vi "Begin.vi"(8 "error in":errorcluster) -> (0 "error out":errorcluster)   [LabVIEW 2017]
doc: "Called before other user functions, this VI is expected to open initial I/O refnums, load in file data, and do all program initialization. Notice that the <B>error out</B> terminal is simply used for data flow. Wiring it to other structures or subVIs ensures that this VI runs first."
uses:
  <vilib>/Rock Robotics/WPI/Solenoid/WPI_SolenoidChannel.ctl
  <vilib>/Rock Robotics/WPI/DriverStation/WPI_DriverStationRobotMode2.ctl
  <vilib>/Rock Robotics/WPI/Joystick/WPI_JoystickDeviceEnum.ctl
  <vilib>/Rock Robotics/SystemInterfaces/spilib/spi_bus.ctl
  Robot Global Data.vi
  <vilib>/Rock Robotics/Network Tables/NT Write String Array.vi
  <vilib>/Rock Robotics/WPI/Solenoid/WPI_SolenoidOpenDouble.vi
  <vilib>/Rock Robotics/WPI/RobotDrive/WPI_RobotDriveOpen4MotorWithExistingMotors.vi
  FIRST-3958-Controls-Library/NavX/navX Library v2/IO/Open/Z900_navX_Open_SPI.vi
  FIRST-3958-Controls-Library/NavX/navX Library v2/navX Library v2.lvlib
panel:
  in  "Reverse Solenoid Channel 2":T1=enum."Solenoid 2"
  in  "Solenoid Channel 2":T1=enum."Solenoid 3"
  in  "Reverse Solenoid Channel":T1
  in  "Solenoid Channel":T1=enum."Solenoid 1"
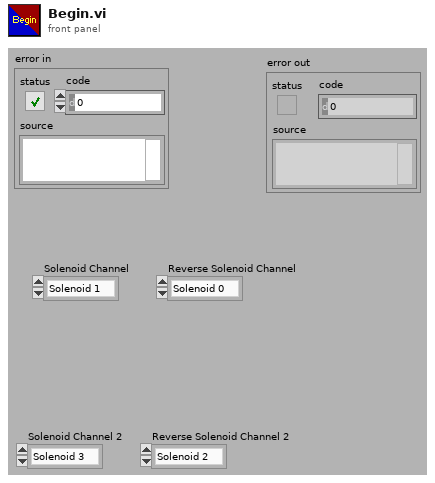
[diagram p1: front panel]
types:
  T1 = typedef "WPI_SolenoidChannel.ctl" = enum8{"Solenoid 0", "Solenoid 1", "Solenoid 2", "Solenoid 3", "Solenoid 4", "Solenoid 5", "Solenoid 6", "Solenoid 7", "Invalid"}
  T2 = typedef "spi_bus.ctl" = enum16{"SPI On-Board, CS0", "SPI On-Board, CS1", "SPI On-Board, CS2", "SPI On-Board, CS3", "SPI MXP", "Invalid"}
  T3 = typedef "WPI_JoystickDeviceEnum.ctl" = enum16{"USB 0", "USB 1", "USB 2", "USB 3", "USB 4", "USB 5"}
  T4 = typedef "WPI_DriverStationRobotMode2.ctl" = enum16{"Autonomous Disabled", "Autonomous Enabled", "Teleop Disabled", "Teleop Enabled", "Disconnected", "Finish", "Test Disabled", "Test Enabled", "Emergency Stopped"}
  T5 = typedef "WPI_MotorControlDeviceRef.ctl" = cluster{"DeviceStatus":errorcluster, "Type":T6, "PWM":cluster{"PWM Channel":T7, "DeadBand":T8}, "CAN":cluster{"Device Number":u8, "SetOutput VI Ref":variant, "GetOutput VI Ref":variant, "Enable VI Ref":variant, "Disable VI Ref":variant, "Data":variant}, "Invert":bool, "DIO PWM":cluster{"PWM \"Enable\" Channel":T7, "DIOChannel":T9, "PWM Rate":dbl}}
  T6 = typedef "WPI_MotorControlType.ctl" = enum16{"PWM", "CAN", "DIO PWM"}
  T7 = typedef "FPGA_DIOPWMChannel.ctl" = enum8{"PWM 0", "PWM 1", "PWM 2", "PWM 3", "PWM 4", "PWM 5", "PWM 6", "PWM 7", "PWM 8", "PWM 9", "PWM MXP 0", "PWM MXP 1", "PWM MXP 2", "PWM MXP 3", "PWM MXP 4", "PWM MXP 5", "PWM MXP 6", "PWM MXP 7", "PWM MXP 8", "PWM MXP 9", "Invalid"}
  T8 = typedef "WPI_PWMDeadband.ctl" = cluster{"Name":string, "maxPositivePwm":i32, "minPositivePwm":i32, "centerPwm":i32, "maxNegativePwm":i32, "minNegativePwm":i32, "angularRange":u16}
  T9 = typedef "FPGA_DIOChannel.ctl" = enum8{"DIO 0", "DIO 1", "DIO 2", "DIO 3", "DIO 4", "DIO 5", "DIO 6", "DIO 7", "DIO 8", "DIO 9", "DIO MXP 0", "DIO MXP 1", "DIO MXP 2", "DIO MXP 3", "DIO MXP 4", "DIO MXP 5", "DIO MXP 6", "DIO MXP 7", "DIO MXP 8", "DIO MXP 9", "DIO MXP 10", "DIO MXP 11", "DIO MXP 12", "DIO MXP 13", "DIO MXP 14", "DIO MXP 15", "SPI Port CS1", "SPI Port CS2", "SPI Port CS3", "SPI Port MISO", "SPI Port MOSI", "Invalid"}
  T10 = typedef "navX Library v2.lvlib/Z900_navX_DeviceTypeDef.ctl" = cluster{"Interface":cluster{"Protocol":T11, "Update Rate (4Hz-100Hz)":u8, "navX Open TypeDef":variant}, "Notify Packet":refnum<notifier>, "Loop VI Refnum":refnum<vi>, "Ready to Close Occurrence Refnum":refnum<k4>}
  T11 = typedef "navX Library v2.lvlib/Z900_navX_ProtocolTypeDef.ctl" = enum16{"SERIAL", "I2C", "SPI"}
  T12 = typedef "WPI_JoystickDevRef.ctl" = cluster{"Device":T3}
  T13 = typedef "WPI_RobotDriveDevRef.ctl" = cluster{"DevStatus":errorcluster, "Motors[]":T5[], "Square Inputs":bool, "Max Output":dbl}
  T14 = typedef "WPI_SolenoidDevRef.ctl" = cluster{"DevStatus":errorcluster, "Pneumatics Control Module":u8, "Forward Solenoid Channel":T1, "Reverse Solenoid Channel":T1}
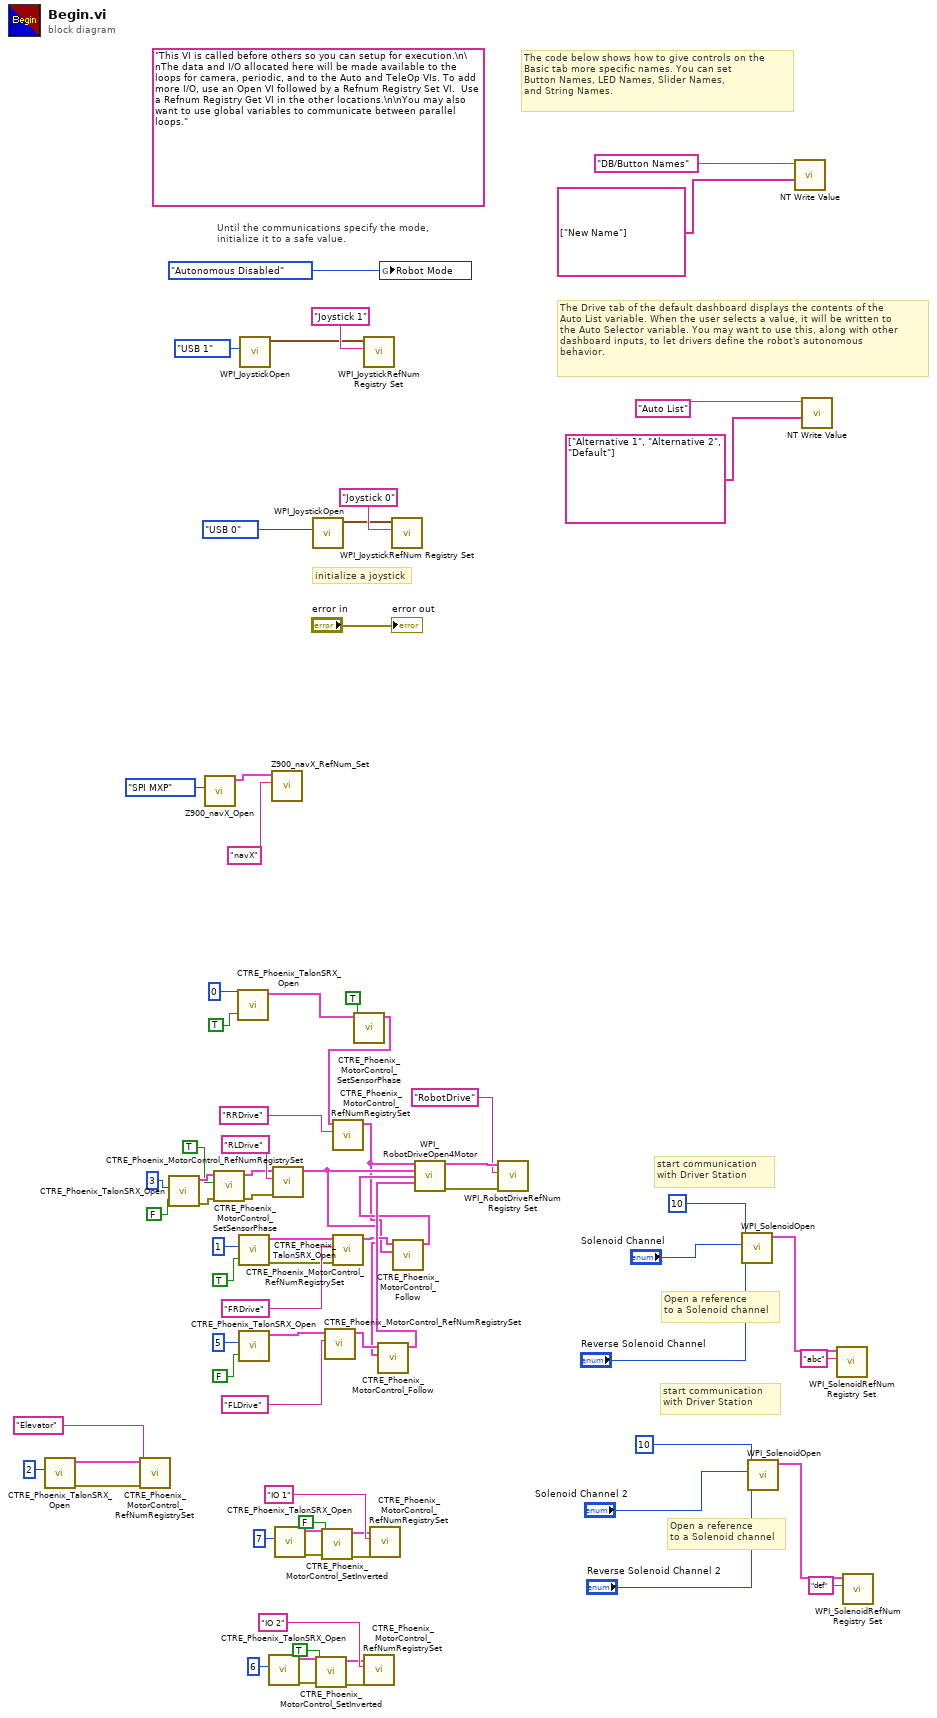
[diagram p0: block diagram]
diagram:
  (unwired) "This VI is called before others so you can setup for execution.\n\nThe data and I/O allocated here will be made available to the loops for camera, periodic, and to the Auto and TeleOp VIs. To add more I/O, use an Open VI followed by a Refnum Registry Set VI.  Use a Refnum Registry Get VI in the other locations.\n\nYou may also want to use global variables to communicate between parallel loops."
  # "start communication with Driver Station"
  # "Open a reference \nto a Solenoid channel"
  # "start communication with Driver Station"
  # "Open a reference \nto a Solenoid channel"
  # "The Drive tab of the default dashboard displays the contents of the\nAuto List variable. When the user selects a value, it will be written to\nthe Auto Selector variable. You may want to use this, along with other\ndashboard inputs, to let drivers define the robot's autonomous\nbehavior."
  # "The code below shows how to give controls on the\nBasic tab more specific names. You can set\nButton Names, LED Names, Slider Names,\nand String Names."
  # "initialize a joystick"
  # "Until the communications specify the mode,\ninitialize it to a safe value."
  n1 = call "CTRE_Phoenix_TalonSRX_Open.vi"("Device Number"=u8 2) -> ("error out"=w50:errorcluster, "CAN Talon SRX Ref"=w49:T5)  [unwired: 9 in]
  n2 = call "CTRE_Phoenix_MotorControl_RefNumRegistrySet.vi"("error in (no error)"=w50, "refnum name"="Elevator", "PhoenixMotorControlDevRef"=w49) -> ()  [unwired: 7 in, 2 out]
  n3 = call "CTRE_Phoenix_TalonSRX_Open.vi"("Invert"=FALSE, "Device Number"=u8 3) -> ("error out"=w44:errorcluster, "CAN Talon SRX Ref"=w46:T5)  [unwired: 8 in]
  n4 = call-poly "Z900_navX_Open.vi"("SPI Bus"=spi_bus."SPI MXP") -> ("navX Device"=w3:T10)  [unwired: 9 in, 1 out]
  n5 = call "CTRE_Phoenix_MotorControl_SetSensorPhase.vi"("error in (no error)"=w44, "PhaseSensor"=TRUE, "PhoenixMotorControlDevRef"=w46) -> ("error out"=w43:errorcluster, "PhoenixMotorControlDevRef"=w45:T5)  [unwired: 7 in]
  n6 = call "CTRE_Phoenix_TalonSRX_Open.vi"("Invert"=TRUE, "Device Number"=u8 0) -> ("CAN Talon SRX Ref"=w11:T5)  [unwired: 8 in, 1 out]
  n7 = call "CTRE_Phoenix_TalonSRX_Open.vi"("Invert"=TRUE, "Device Number"=u8 1) -> ("error out"=w12:errorcluster, "CAN Talon SRX Ref"=w13:T5)  [unwired: 8 in]
  n8 = call "CTRE_Phoenix_TalonSRX_Open.vi"("Invert"=FALSE, "Device Number"=u8 5) -> ("CAN Talon SRX Ref"=w52:T5)  [unwired: 8 in, 1 out]
  n9 = call <vilib>:"WPI_JoystickOpen.vi"("JoystickDevice"=WPI_JoystickDeviceEnum."USB 1") -> ("JoystickDevRef"=w35:T12)  [unwired: 10 in]
  n10 = call "CTRE_Phoenix_TalonSRX_Open.vi"("Device Number"=u8 6) -> ("error out"=w23:errorcluster, "CAN Talon SRX Ref"=w26:T5)  [unwired: 9 in]
  n11 = call "Z900_navX_RefNum_Set.vi"("refnum name"="navX", "navX Device"=w3) -> ()  [unwired: 8 in, 2 out]
  n12 = call "CTRE_Phoenix_MotorControl_RefNumRegistrySet.vi"("error in (no error)"=w43, "refnum name"="RLDrive", "PhoenixMotorControlDevRef"=w45) -> ("PhoenixMotorControlDevRef"=w7:T5)  [unwired: 7 in, 1 out]
  n13 = call "CTRE_Phoenix_TalonSRX_Open.vi"("Device Number"=u8 7) -> ("error out"=w29:errorcluster, "CAN Talon SRX Ref"=w32:T5)  [unwired: 9 in]
  n14 = call <vilib>:"WPI_JoystickOpen.vi"("JoystickDevice"=WPI_JoystickDeviceEnum."USB 0") -> ("JoystickDevRef"=w73:T12)  [unwired: 10 in]
  n15 = call "CTRE_Phoenix_MotorControl_SetInverted.vi"("error in (no error)"=w23, "Invert?"=TRUE, "PhoenixMotorControlDevRef"=w26) -> ("error out"=w22:errorcluster, "PhoenixMotorControlDevRef"=w25:T5)  [unwired: 7 in]
  n16 = call "CTRE_Phoenix_MotorControl_SetInverted.vi"("error in (no error)"=w29, "Invert?"=FALSE, "PhoenixMotorControlDevRef"=w32) -> ("error out"=w28:errorcluster, "PhoenixMotorControlDevRef"=w31:T5)  [unwired: 7 in]
  n17 = call "CTRE_Phoenix_MotorControl_RefNumRegistrySet.vi"("refnum name"="FLDrive", "PhoenixMotorControlDevRef"=w52) -> ("PhoenixMotorControlDevRef"=w9:T5)  [unwired: 8 in, 1 out]
  n18 = call "CTRE_Phoenix_MotorControl_RefNumRegistrySet.vi"("error in (no error)"=w12, "refnum name"="FRDrive", "PhoenixMotorControlDevRef"=w13) -> ("PhoenixMotorControlDevRef"=w6:T5)  [unwired: 7 in, 1 out]
  n19 = call "CTRE_Phoenix_MotorControl_SetSensorPhase.vi"("PhaseSensor"=TRUE, "PhoenixMotorControlDevRef"=w11) -> ("PhoenixMotorControlDevRef"=w10:T5)  [unwired: 8 in, 1 out]
  n20 = call "CTRE_Phoenix_MotorControl_RefNumRegistrySet.vi"("refnum name"="RRDrive", "PhoenixMotorControlDevRef"=w10) -> ("PhoenixMotorControlDevRef"=w4:T5)  [unwired: 8 in, 1 out]
  n21 = call <vilib>:"WPI_JoystickRefNum Registry Set.vi"("refnum name"="Joystick 1", "JoystickDevRef"=w35) -> ()  [unwired: 8 in, 2 out]
  n22 = call "CTRE_Phoenix_MotorControl_RefNumRegistrySet.vi"("error in (no error)"=w22, "refnum name"="IO 2", "PhoenixMotorControlDevRef"=w25) -> ()  [unwired: 7 in, 2 out]
  n23 = call "CTRE_Phoenix_MotorControl_RefNumRegistrySet.vi"("error in (no error)"=w28, "refnum name"="IO 1", "PhoenixMotorControlDevRef"=w31) -> ()  [unwired: 7 in, 2 out]
  n24 = call "CTRE_Phoenix_MotorControl_Follow.vi"("Master Controller to Follow"=w7, "PhoenixMotorControlDevRef"=w9) -> ("PhoenixMotorControlDevRef"=w8:T5)  [unwired: 8 in, 1 out]
  n25 = global write "Robot Global Data.vi" "Robot Mode"(WPI_DriverStationRobotMode2."Autonomous Disabled" ("Robot Mode")) -> ()
  n26 = call <vilib>:"WPI_JoystickRefNum Registry Set.vi"("refnum name"="Joystick 0", "JoystickDevRef"=w73) -> ()  [unwired: 8 in, 2 out]
  n27 = call "CTRE_Phoenix_MotorControl_Follow.vi"("Master Controller to Follow"=w4, "PhoenixMotorControlDevRef"=w6) -> ("PhoenixMotorControlDevRef"=w5:T5)  [unwired: 8 in, 1 out]
  n28 = call-poly <vilib>:"WPI_RobotDriveOpen4Motor.vi"("Rear Left Motor Dev Ref"=w4, "Rear Right Motor Dev Ref"=w7, "Front Left Motor Dev Ref"=w5, "Front Right Motor Dev Ref"=w8) -> ("RobotDriveDevRef"=w61:T13, "error out"=w62:errorcluster)  [unwired: 10 in]
  n29 = call <vilib>:"WPI_RobotDriveRefNum Registry Set.vi"("error in (no error)"=w62, "refnum name"="RobotDrive", "RobotDriveDevRef"=w61) -> ()  [unwired: 7 in, 2 out]
  n30 = call-poly <vilib>:"WPI_SolenoidOpen.vi"("Reverse Solenoid Channel"="Reverse Solenoid Channel", "Forward Solenoid Channel"="Solenoid Channel", "Pneumatics Control Module (0)"=u8 10) -> ("SolenoidDevRef"=w39:T14)  [unwired: 1 in, 7 out]
  n31 = call-poly <vilib>:"WPI_SolenoidOpen.vi"("Reverse Solenoid Channel"="Reverse Solenoid Channel 2", "Forward Solenoid Channel"="Solenoid Channel 2", "Pneumatics Control Module (0)"=u8 10) -> ("SolenoidDevRef"=w18:T14)  [unwired: 1 in, 7 out]
  n32 = call-poly <vilib>:"NT Write Value.vi"("String Array"=string[] ["New Name"], "Name"="DB/Button Names") -> ()  [unwired: 9 in, 1 out]
  n33 = call-poly <vilib>:"NT Write Value.vi"("String Array"=string[] ["Alternative 1", "Alternative 2", "Default"], "Name"="Auto List") -> ()  [unwired: 9 in, 1 out]
  n34 = call <vilib>:"WPI_SolenoidRefNum Registry Set.vi"("refnum name"="abc", "SolenoidDevRef"=w39) -> ()  [unwired: 8 in, 2 out]
  n35 = call <vilib>:"WPI_SolenoidRefNum Registry Set.vi"("refnum name"="def", "SolenoidDevRef"=w18) -> ()  [unwired: 8 in, 2 out]
  "error out" <- "error in"
